vi "EfficientTurnMath.vi"(8 "current":dbl format="%#_13g", 11 "target":dbl format="%#_13g") -> (0 "Invert":bool, 3 "AngleToTurn":dbl)   [LabVIEW 2020]
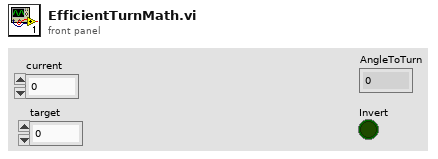
[diagram p1: front panel]
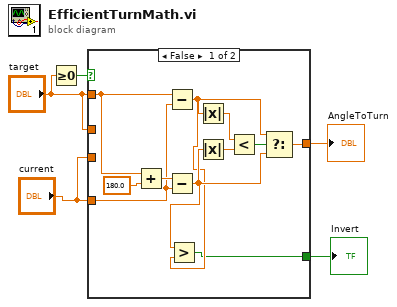
[diagram p0: block diagram]
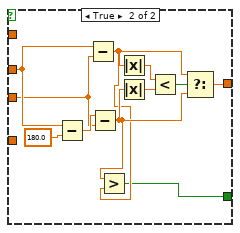
[diagram p2: hidden frame]
diagram:
  n1 = Greater Or Equal To 0?(x="target") -> (x >= 0?=w5:bool)
  n2 = case shown="False" w5 {
    tunnel: "target" -> [_ w22]
    tunnel: "target" -> [w12 _]
    tunnel: [w11 w21] -> w3
    tunnel: "current" -> [w9 _]
    tunnel: "current" -> [_ w20]
    tunnel: [w6 w17] -> w1
    frame False {
      n3 = Add(x=w12, y=180.0) -> (x+y=w13:dbl)
      n4 = Subtract(x=w12, y=w9) -> (x-y=w7:dbl)
      n5 = Subtract(x=w13, y=w9) -> (x-y=w8:dbl)
      n6 = Greater?(x=w8, y=w7) -> (0:w6:bool)
      n7 = Absolute Value(x=w7) -> (abs(x)=w10:dbl)
      n8 = Absolute Value(x=w8) -> (abs(x)=w14:dbl)
      n9 = Less?(x=w10, y=w14) -> (x < y?=w15:bool)
      n10 = Select(t=w7, s=w15, f=w8) -> (s? t:f=w11:dbl)
    }
    frame True {
      n11 = Subtract(x=w22, y=180.0) -> (x-y=w23:dbl)
      n12 = Subtract(x=w22, y=w20) -> (x-y=w18:dbl)
      n13 = Subtract(x=w23, y=w20) -> (x-y=w19:dbl)
      n14 = Greater?(x=w19, y=w18) -> (0:w17:bool)
      n15 = Absolute Value(x=w18) -> (abs(x)=w25:dbl)
      n16 = Absolute Value(x=w19) -> (abs(x)=w24:dbl)
      n17 = Less?(x=w25, y=w24) -> (x < y?=w26:bool)
      n18 = Select(t=w18, s=w26, f=w19) -> (s? t:f=w21:dbl)
    }
  }
  "AngleToTurn" <- w3
  "Invert" <- w1
